vi "8 PulseMeasurements f+DC.vi"(2 "8 PulseMeas Chs":bool[](array[boolean])=[FALSE, FALSE, FALSE, FALSE, FALSE, FALSE, FALSE, FALSE], 4 "PulseMeas Timeouts":u32[](array[numeric])=[0, 0, 0, 0, 0, 0, 0, 0]) -> (7 "PulseMeas Packets DC-f":u64[](array[numeric]))   [LabVIEW 2014]
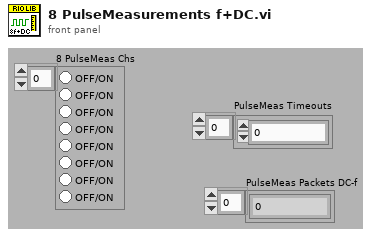
[diagram p1: front panel]
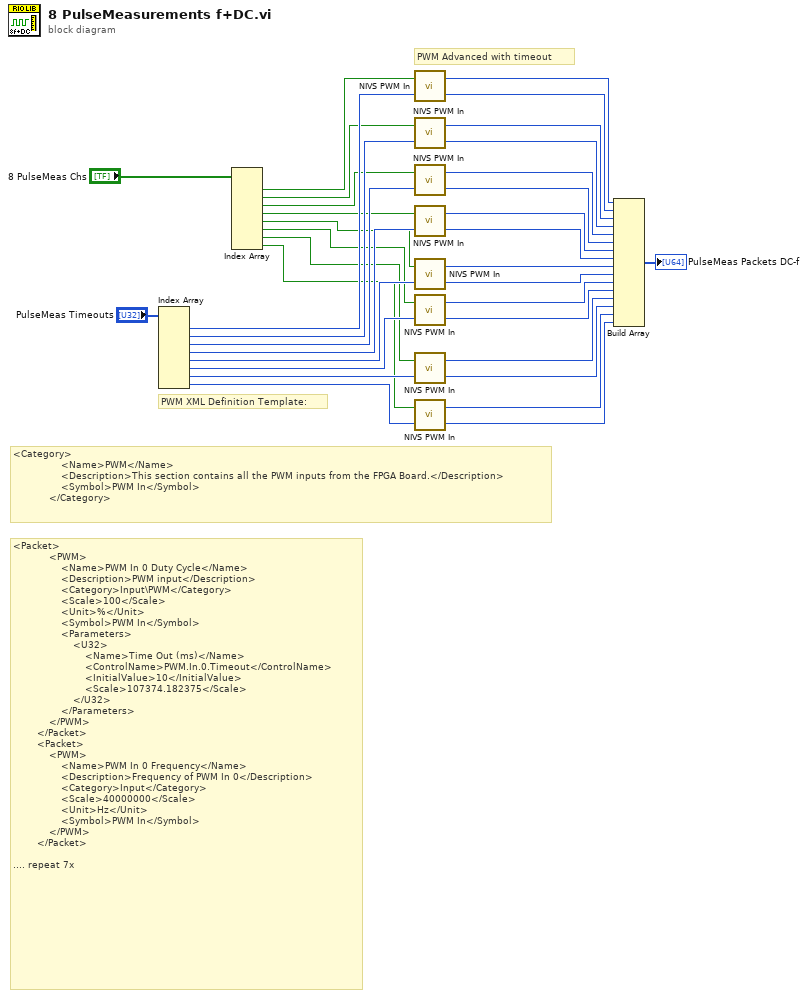
[diagram p0: block diagram]
diagram:
  # "<Category>\n                <Name>PWM</Name>\n                <Description>This section contains all the PWM inputs from the FPGA Board.</Description>\n                <Symbol>PWM In</Symbol>\n            </Category>"
  # "PWM XML Definition Template:"
  # "<Packet>\n            <PWM>\n                <Name>PWM In 0 Duty Cycle</Name>\n                <Description>PWM input</Description>\n                <Category>Input\\PWM</Category>\n                <Scale>100</Scale>\n                <Unit>%</Unit>\n                <Symbol>PWM In</Symbol>\n                <Parameters>\n                    <U32>\n                        <Name>Time Out (ms)</Name>\n                        <ControlName>PWM.In.0.Timeout</ControlName>\n                        <InitialValue>10</InitialValue>\n                        <Scale>107374.182375</Scale>\n                    </U32>\n                </Parameters>\n            </PWM>\n        </Packet>\n        <Packet>\n            <PWM>\n                <Name>PWM In 0 Frequency</Name>\n                <Description>Frequency of PWM In 0</Description>\n                <Category>Input</Category>\n                <Scale>40000000</Scale>\n                <Unit>Hz</Unit>\n                <Symbol>PWM In</Symbol>\n            </PWM>\n        </Packet>\n\n.... repeat 7x"
  # "PWM Advanced with timeout"
  n1 = Index Array(array="PulseMeas Timeouts") -> (element #1=w27:u32, element #2=w28:u32, element #3=w29:u32, element #4=w30:u32, element #5=w31:u32, element #6=w32:u32, element #7=w33:u32, element #8=w34:u32)  [unwired: 8 in]
  n2 = Index Array(array="8 PulseMeas Chs") -> (element #1=w26:bool, element #2=w8:bool, element #3=w7:bool, element #4=w6:bool, element #5=w5:bool, element #6=w4:bool, element #7=w3:bool, element #8=w2:bool)  [unwired: 8 in]
  n3 = call "NIVS PWM In.vi"("PWM In Timeout"=w27, "DI"=w26) -> ("PWM In Freq Packet"=w24:u64, "PWM In DC Packet"=w25:u64)
  n4 = call "NIVS PWM In.vi"("PWM In Timeout"=w28, "DI"=w8) -> ("PWM In Freq Packet"=w22:u64, "PWM In DC Packet"=w23:u64)
  n5 = call "NIVS PWM In.vi"("PWM In Timeout"=w29, "DI"=w7) -> ("PWM In Freq Packet"=w20:u64, "PWM In DC Packet"=w21:u64)
  n6 = call "NIVS PWM In.vi"("PWM In Timeout"=w30, "DI"=w6) -> ("PWM In Freq Packet"=w18:u64, "PWM In DC Packet"=w19:u64)
  n7 = call "NIVS PWM In.vi"("PWM In Timeout"=w31, "DI"=w5) -> ("PWM In Freq Packet"=w16:u64, "PWM In DC Packet"=w17:u64)
  n8 = call "NIVS PWM In.vi"("PWM In Timeout"=w32, "DI"=w4) -> ("PWM In Freq Packet"=w14:u64, "PWM In DC Packet"=w15:u64)
  n9 = call "NIVS PWM In.vi"("PWM In Timeout"=w33, "DI"=w3) -> ("PWM In Freq Packet"=w12:u64, "PWM In DC Packet"=w13:u64)
  n10 = call "NIVS PWM In.vi"("PWM In Timeout"=w34, "DI"=w2) -> ("PWM In Freq Packet"=w10:u64, "PWM In DC Packet"=w11:u64)
  n11 = Build Array(w25, w24, w23, w22, w21, w20, w19, w18, w17, w16, w15, w14, w13, w12, w11, w10) -> (→"PulseMeas Packets DC-f":u64[])
